vi "seatLeakageTest.vi"(7 "LabVIEW Web Service Request":refnum<class "Web Request.lvclass">, 9 "unit":dbl, 10 "testPressure":dbl, 11 "time":dbl) -> (2 "startingPressure":dbl format="%#_2g", 3 "finalPressure":dbl)   [LabVIEW 2015]
uses:
  <vilib>/wsapi/Web Request.lvclass
  <vilib>/Waveform/WDTOps.llb/WDT Append Waveforms DBL.vi
panel:
  in  "Stop (Pressure Reading)":bool
  out "data":waveform(dbl)[](graph)
  out "timer":dbl
  in  "Stop timer":bool
  in  "Start timer":bool
  out "value":string
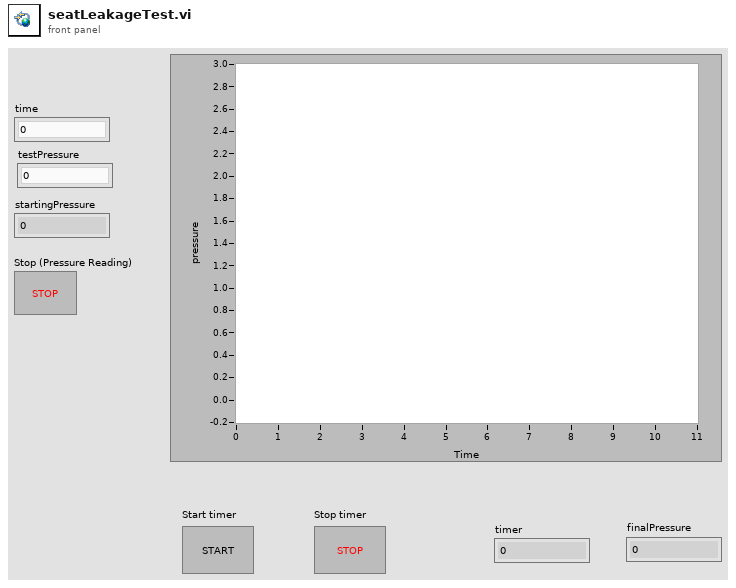
[diagram p1: front panel]
types:
  T1 = typedef "imagedata.ctl" = cluster{"image type":i32, "image depth":i32, "image":u8[], "mask":u8[], "colors":u32[], "Rectangle":cluster{"left":i16, "top":i16, "right":i16, "bottom":i16}}
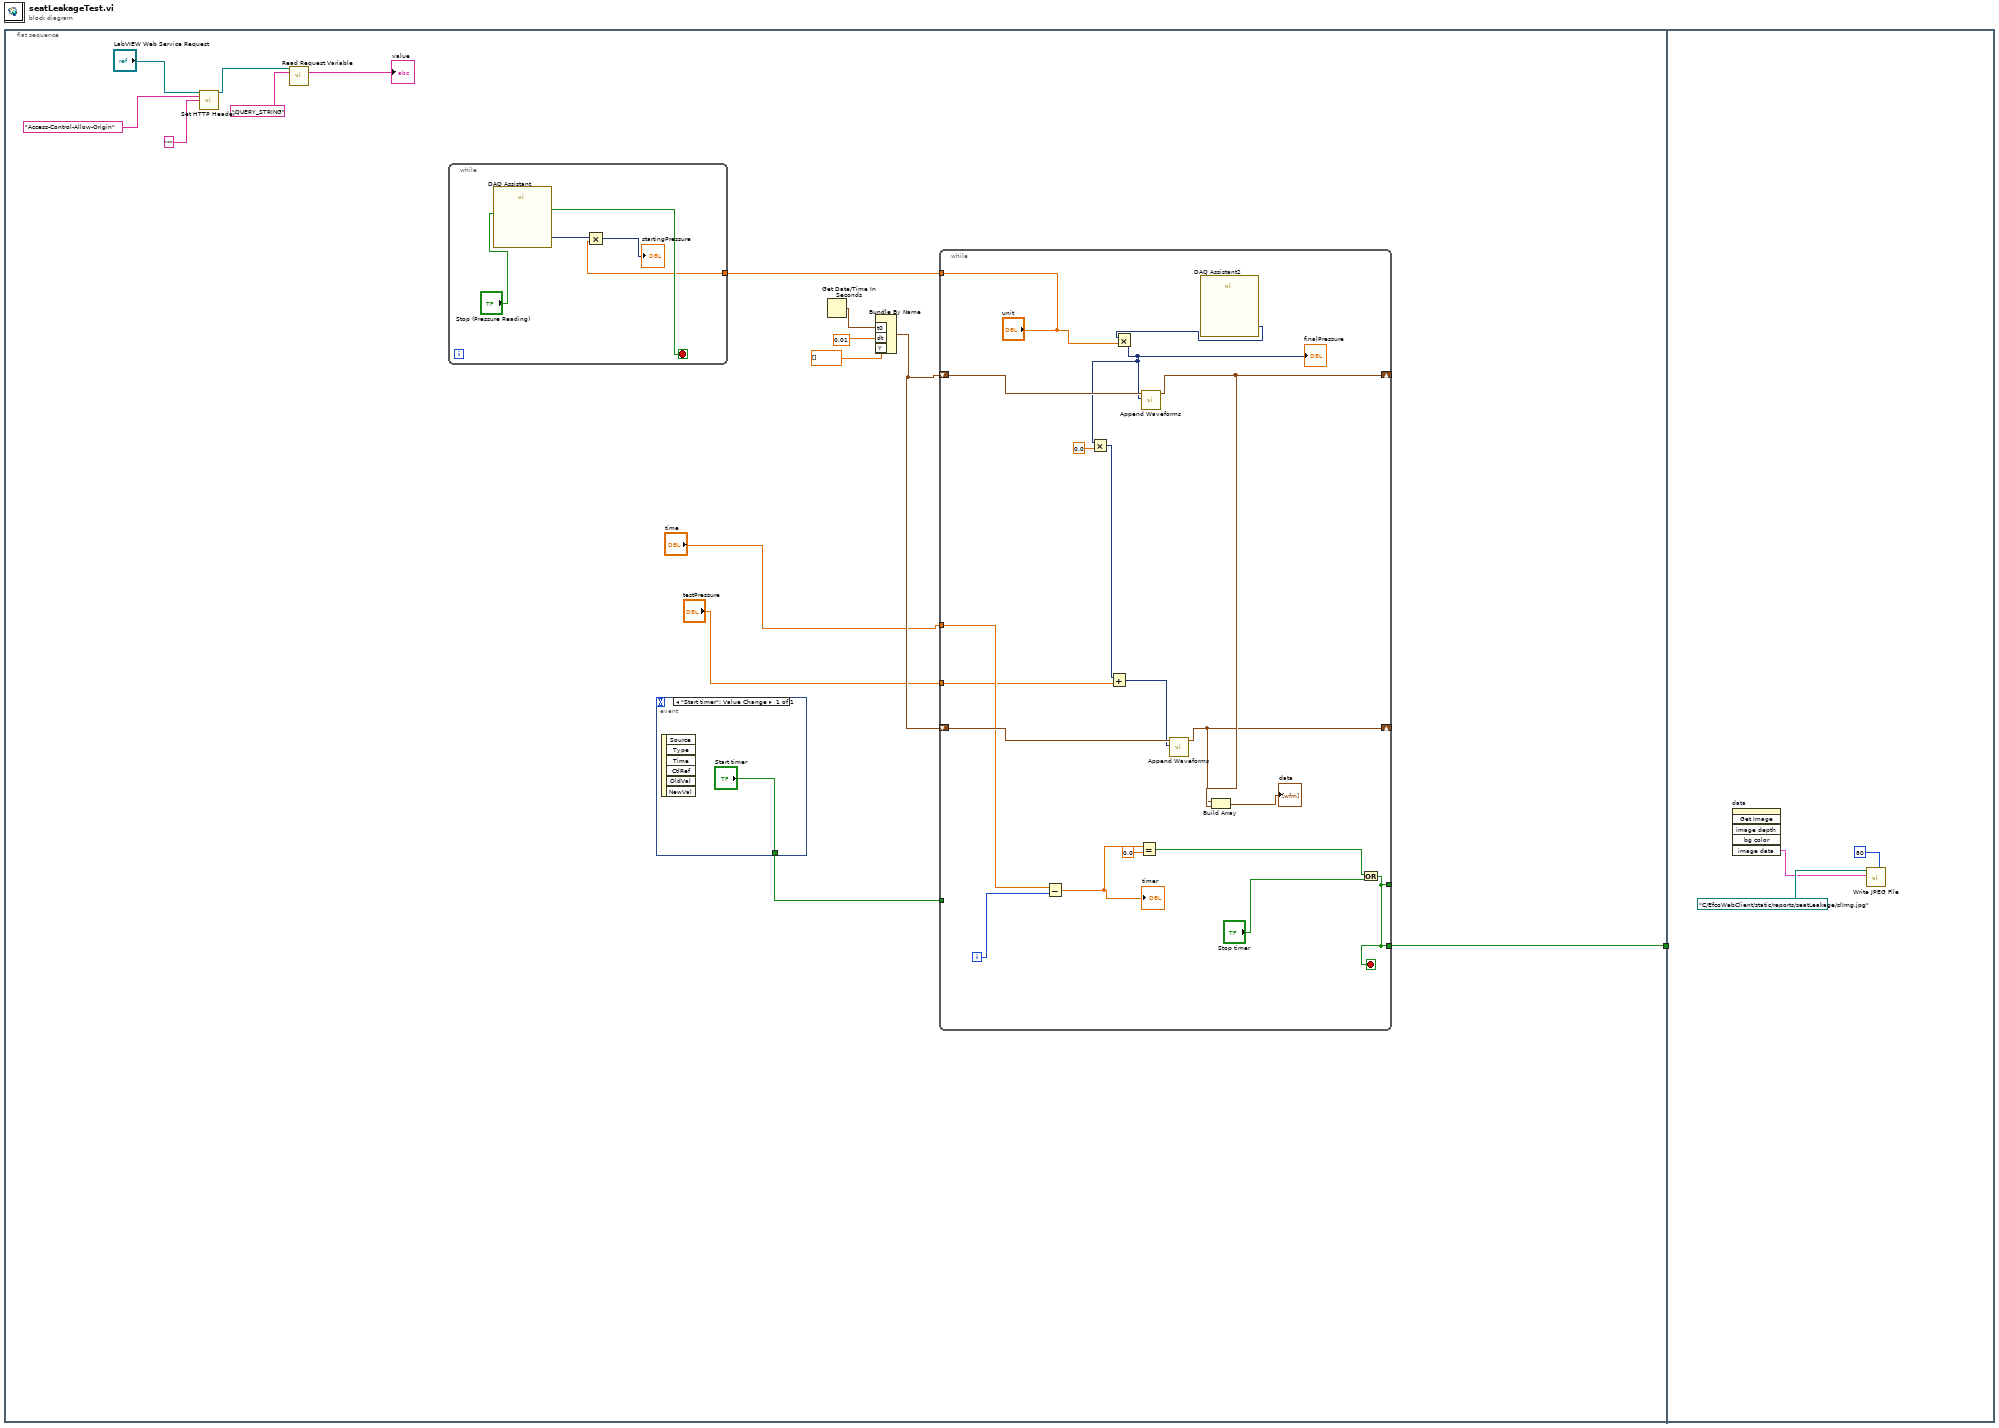
[diagram p0: block diagram]
diagram:
  n1 = flat-sequence {
    tunnel: [w9] -> w1
    tunnel: w1 -> [_]
    frame #0 {
      n2 = call <vilib>:"Set HTTP Header.vi"("LabVIEW Web Service Request"="LabVIEW Web Service Request", "header"="Access-Control-Allow-Origin", "header value"="*") -> ("LabVIEW Web Service Request out"=w5:refnum<class "Web Request.lvclass">)  [unwired: 11 in, 1 out]
      n3 = call <vilib>:"Read Request Variable.vi"("LabVIEW Web Service Request"=w5, "variable name"="QUERY_STRING") -> ("value"=→"value":string)  [unwired: 11 in, 2 out]
      n4 = event shown="[0] \"Start timer\": Value Change" {
        selector: _ -> [_]
        dyn-events: _ -> [_]
        timeout: _ -> [_]
        tunnel: ["Start timer"] -> w13
        event "Start timer": Value Change {
          n5 = event-data() -> ()  [unwired: 1 in, 6 out]
        }
      }
      n6 = Get Date/Time In Seconds() -> (seconds since 1Jan1904=w16:timestamp)
      n7 = Bundle By Name("t0"=w16, "dt"=0.01, "Y"=dbl[] []) -> (w12:waveform(dbl))  [unwired: 1 in]
      n8 = while {
        shift-right: [w31] -> _
        shift-left: w12 -> [w36]
        tunnel: "time" -> [w27]
        shift-right: [w30] -> _
        shift-left: w12 -> [w35]
        tunnel: w13 -> [_]
        tunnel: "testPressure" -> [w21]
        tunnel: [w19] -> w9
        tunnel: [w19] -> _
        tunnel: ["unit"] -> w2
        i -> [w28]
        stop <- w19 stop-if-true
        n9 = Subtract(x=w27, y=w28) -> (x-y=w26:dbl)
        "timer" <- w26
        n10 = Equal?(x=w26, y=0.0) -> (x = y?=w24:bool)
        n11 = call "DAQ Assistant2"() -> ("data"=w29:dynamicdata)  [unwired: 16 in, 3 out]
        n12 = Multiply(x=w29, y="unit") -> (x*y=w34:dynamicdata)
        "finalPressure" <- w34
        n13 = Multiply(x=w34, y=0.0) -> (x*y=w32:dynamicdata)
        n14 = Add(x=w32, y=w21) -> (x+y=w22:dynamicdata)
        n15 = call-poly <vilib>:"Append Waveforms.vi"("waveform B"=w34, "waveform A"=w36) -> ("waveform out"=w31:waveform(dbl))  [unwired: 8 in, 1 out]
        n16 = call-poly <vilib>:"Append Waveforms.vi"("waveform B"=w22, "waveform A"=w35) -> ("waveform out"=w30:waveform(dbl))  [unwired: 8 in, 1 out]
        n17 = Build Array(w30, w31) -> (→"data":waveform(dbl)[])
        n18 = Or(x=w24, y="Stop timer") -> (x .or. y?=w19:bool)
      }
      n19 = while {
        tunnel: w2 -> [w37]
        stop <- w38 stop-if-true
        n20 = call "DAQ Assistant"("stop (F)"="Stop (Pressure Reading)") -> ("data"=w41:dynamicdata, "stopped"=w38:bool)  [unwired: 15 in, 2 out]
        n21 = Multiply(x=w41, y=w37) -> (x*y=→"startingPressure":dynamicdata)
      }
    }
    frame #1 {
      n22 = invoke on="data" class="WFGraph (strict)" method="Get Image"() -> ("image data"=w43:T1)  [unwired: 6 in, 5 out]
      n23 = call <vilib>:"Write JPEG File.vi"("quality (80)"=80, "image data"=w43, "path to JPEG file"=path "C:/EfcoWebClient/static/reports/seatLeakage/slImg.jpg") -> ()  [unwired: 7 in, 2 out]
    }
  }
